vi "Data.vi"(11 "Error Msg Strategy in":refnum<class "Error Msg.lvclass">) -> (2 "Error":errorcluster)   [LabVIEW 2021, in "Error.lvlib" / "Error Msg.lvclass"]
uses:
  Error Msg.lvclass
  Error Msg.lvclass/Error Msg.ctl
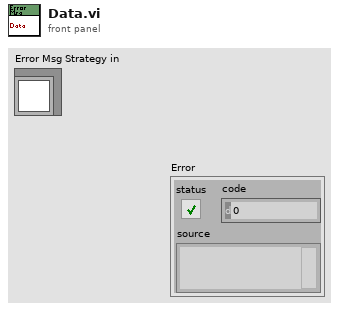
[diagram p1: front panel]
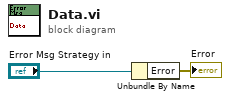
[diagram p0: block diagram]
diagram:
  n1 = Unbundle By Name("Error Msg Strategy in") -> ("Error"=→"Error":errorcluster)
